vi "varshni fit function - 5par.vi"(3 "output control":T1, 4 "data":T2, 5 "X":dbl[](array[numeric]), 6 "a":dbl[](array[numeric])) -> (0 "error out":errorcluster, 1 "f'(X,a)":dbl[][](array[numeric]), 2 "f(X,a)":dbl[](array[numeric]))   [LabVIEW 2010]
doc: "This template is the starting point for creating a model function to be passed to the Nonlinear Curve Fit.vi."
uses:
  <vilib>/gmath/NumericalOptimization/objective function data.ctl
  <vilib>/gmath/NumericalOptimization/LM_output select.ctl
  <vilib>/gmath/NI_Gmath.lvlib
panel:
  in  "fit":enum16{"other", "3par", "5par"}(ring)=enum."3par"
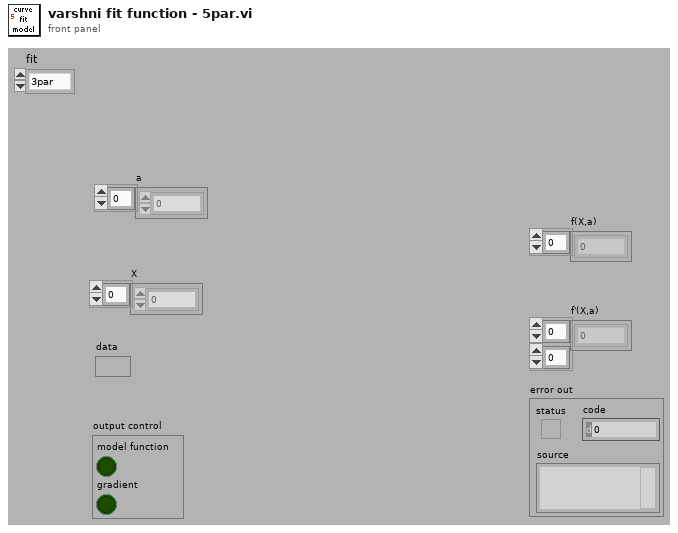
[diagram p1: front panel]
types:
  T1 = typedef "NI_Gmath.lvlib/LM_output select.ctl" = cluster{"model function":bool, "gradient":bool}
  T2 = typedef "NI_Gmath.lvlib/objective function data.ctl" = variant
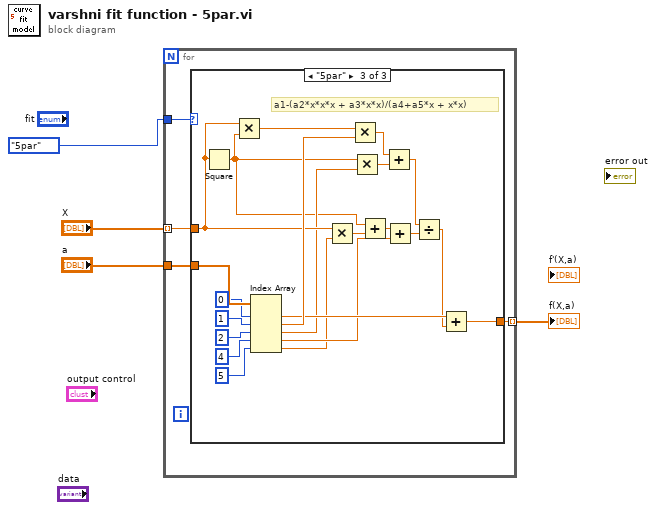
[diagram p0: block diagram]
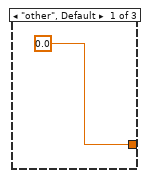
[diagram p2: hidden frame]
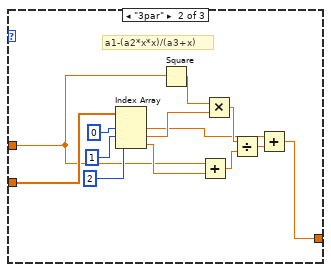
[diagram p3: hidden frame]
diagram:
  n1 = for {
    tunnel: "a" -> [w8]
    tunnel: "X" -> [w6] mode=indexing
    tunnel: [w7] -> w2 mode=indexing
    tunnel: enum16{"other", "3par", "5par"}."5par" ("action") -> [w5]
    n2 = case shown="\"5par\"" w5 {
      tunnel: w8 -> [_ w22 w44]
      tunnel: [0.0 w12 w36] -> w7
      tunnel: w6 -> [_ w11 w32]
      frame "other", Default {
      }
      frame "3par" {
        # "a1-(a2*x*x)/(a3+x)"
        n3 = Index Array(array=w22, index #1=0 ("index"), index #2=1 ("index"), index #3=2 ("index")) -> (element #1=w14:dbl, element #2=w18:dbl, element #3=w17:dbl)
        n4 = Square(x=w11) -> (x^2=w10:dbl)
        n5 = Add(x=w11, y=w17) -> (x+y=w15:dbl)
        n6 = Multiply(x=w10, y=w18) -> (x*y=w16:dbl)
        n7 = Divide(x=w16, y=w15) -> (x/y=w13:dbl)
        n8 = Add(x=w14, y=w13) -> (x+y=w12:dbl)
      }
      frame "5par" {
        # "a1-(a2*x*x*x + a3*x*x)/(a4+a5*x + x*x)"
        n9 = Square(x=w32) -> (x^2=w26:dbl)
        n10 = Multiply(x=w32, y=w26) -> (x*y=w28:dbl)
        n11 = Index Array(array=w44, index #1=0 ("index"), index #2=1 ("index"), index #3=2 ("index"), index #4=4 ("index"), index #5=5 ("index")) -> (element #1=w38:dbl, element #2=w40:dbl, element #3=w27:dbl, element #4=w33:dbl, element #5=w31:dbl)
        n12 = Multiply(x=w32, y=w31) -> (x*y=w30:dbl)
        n13 = Multiply(x=w28, y=w40) -> (x*y=w24:dbl)
        n14 = Multiply(x=w26, y=w27) -> (x*y=w25:dbl)
        n15 = Add(x=w26, y=w30) -> (x+y=w29:dbl)
        n16 = Add(x=w24, y=w25) -> (x+y=w23:dbl)
        n17 = Add(x=w29, y=w33) -> (x+y=w39:dbl)
        n18 = Divide(x=w23, y=w39) -> (x/y=w37:dbl)
        n19 = Add(x=w38, y=w37) -> (x+y=w36:dbl)
      }
    }
  }
  "f(X,a)" <- w2
